vi "Acquire stream and Plot.vi"(6 "method":T1={"sampling interval"=0.1, "samples to average"=1, "data interval"=0.0, "stream data"=FALSE, "file path"=refnum, "command"={"command"=enum."Idle", "start time (ms)"=0, "Channel Indices"=[], "Scans per Sample"=1}} {"command"."Scans per Sample" min=1; "data interval" format="%.2f"; "samples to average" min=1 step=1; "sampling interval" format="%.2f"}, 8 "Reset":bool, 9 "history length":u16, 10 "Log Data":bool, 11 "connection ID":refnum<k5>) -> (0 "Status":bool, 3 "Multiplot graph data":cluster{dbl[], dbl[]}[](array[cluster]) {"?" format="%.2f"; "?" format="%.2f"})   [LabVIEW 2010]
uses:
  DataServer/command.ctl
  DataServer/command cluster.ctl
  DAC apps/support/method.ctl
panel:
  # "s"
  # "s"
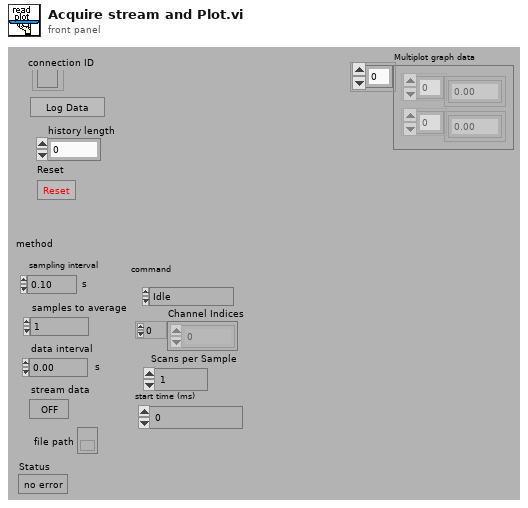
[diagram p1: front panel]
types:
  T1 = typedef "method.ctl" = cluster{"sampling interval":sgl, "samples to average":u32, "data interval":sgl, "stream data":bool, "file path":refnum<file>, "command":T2}
  T2 = typedef "command cluster.ctl" = cluster{"command":T3, "start time (ms)":u32, "Channel Indices":i32[], "Scans per Sample":i32}
  T3 = typedef "command.ctl" = enum16{"Idle", "Send Data", "Send 1 Scan", "Logoff"}
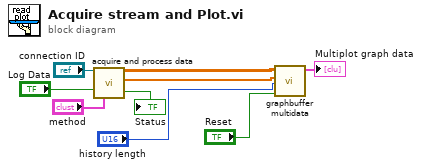
[diagram p0: block diagram]
diagram:
  n1 = call "acquire and process data.vi"("connection ID"="connection ID", "Log Data"="Log Data", "method"="method") -> ("data out"=w8:sgl[][], "Time"=w7:dbl[], "Status"=→"Status":bool)  [unwired: 5 in, 5 out]
  n2 = call <userlib>:"graphbuffer multidata.vi"("Reset"="Reset", "history length"="history length", "Time"=w7, "data"=w8) -> ("Multiplot graph data"=→"Multiplot graph data":cluster{dbl[], dbl[]}[])  [unwired: 5 in, 2 out]
